vi "PH_ImageCalibrator.ProcPeriodic.vi"(0 "i ref in":refnum<vi>, 3 "ms timeout (100)":i32=100, 5 "error in (no error)":errorcluster) -> (14 "i ref out":refnum<vi>, 17 "timed out":bool, 19 "error out":errorcluster)   [LabVIEW 2014, in "PH_ImageCalibrator.lvlib"]
doc: "This method serves to periodically do things like reading values from the HW. Methods that should be executed periodically should be called from THIS methode. Add code here."
uses:
  PH_ImageCalibrator.lvlib
  PH_Basics/PH_Img_BaseClass/PH_Img_BaseClass.lvlib
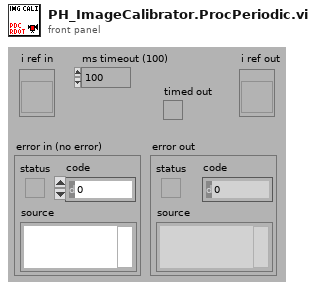
[diagram p1: front panel]
types:
  T1 = typedef "PH_Img_BaseClass.lvlib/PH_Img_BaseClass.i attribute.ctl" = cluster{"GUI Refs":T2, "Timeout Image [ms]":i32, "Default Periodic Period [ms]":i32, "Camera":cluster{"Instancename":string, "Notifier":refnum<notifier>}, "Palette":T3, "Cam Settings":cluster{"Cam ID":string, "Gain":dbl, "Brightness":dbl, "Shutter":dbl, "Cam Info Failure":bool, "Mode":i32}}
  T2 = typedef "PH_Img_BaseClass.lvlib/PH_Img_BaseClass.GUI Refs.ctl" = cluster{"Timeout":refnum<vi>, "Image":refnum<vi>, "Palette":refnum<vi>, "Timeout Set":refnum<vi>}
  T3 = typedef "PH_Img_BaseClass.lvlib/PH_Img_BaseClass.Palette.ctl" = i32
  T4 = typedef "IMAQ Image.ctl" = refnum<image>
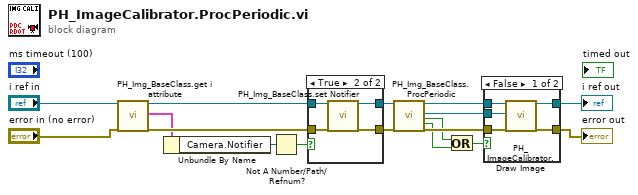
[diagram p0: block diagram]
diagram:
  n1 = call "PH_Img_BaseClass.get i attribute.vi"("i ref in"="i ref in", "error in (no error)"="error in (no error)") -> ("i ref out"=w12:refnum<vi>, "i attribute"=w14:T1, "error out"=w15:errorcluster)  [unwired: 15 in]
  n2 = Unbundle By Name(w14) -> ("Camera.Notifier"=w10:refnum<notifier>)
  n3 = Not A Number/Path/Refnum?(number/path/refnum=w10) -> (NaN/Path/Refnum?=w11:bool)
  n4 = case shown="True" w11 {
    tunnel: w15 -> [w19 w20]
    tunnel: w12 -> [w18 w23]
    tunnel: [w18 w22] -> w7
    tunnel: [w19 w21] -> w6
    frame False {
    }
    frame True {
      n5 = call "PH_Img_BaseClass.set Notifier.vi"("i ref in"=w23, "error in"=w20) -> ("i ref out"=w22:refnum<vi>, "error out"=w21:errorcluster)  [unwired: 16 in]
    }
  }
  n6 = call "PH_Img_BaseClass.ProcPeriodic.vi"("i ref in"=w7, "error in (no error)"=w6) -> ("i ref out"=w8:refnum<vi>, "Cam Image"=w9:T4, "timed out?"=w3:bool, "Error while unflatten data?"=w2:bool, "error out"=w5:errorcluster)  [unwired: 13 in]
  n7 = Or(x=w3, y=w2) -> (x .or. y?=w1:bool)
  n8 = case shown="False" w1 {
    tunnel: w8 -> [w28 w30]
    tunnel: [w25 w30] -> w13
    tunnel: w5 -> [w27 w29]
    tunnel: [w26 w29] -> w4
    tunnel: w9 -> [w24 _]
    frame False {
      n9 = call "PH_ImageCalibrator.Draw Image.vi"("i ref in"=w28, "Cam Image"=w24, "error in (no error)"=w27) -> ("i ref out"=w25:refnum<vi>, "error out"=w26:errorcluster)  [unwired: 15 in]
    }
    frame True {
    }
  }
  "error out" <- w4
  "i ref out" <- w13
